vi "Overview Mouse Down.vi"(8 "error in":errorcluster, 10 "Coords":T1, 11 "XYGraphOverview in":refnum<class "XYGraphOverview.lvclass">) -> (0 "error out":errorcluster, 3 "XYGraphOverview out":refnum<class "XYGraphOverview.lvclass">)   [LabVIEW 2020, in "XYGraphOverview.lvlib" / "XYGraphOverview.lvclass"]
uses:
  XYGraphOverview.lvclass
  <vilib>/Utility/miscctls.llb/LVPoint32TypeDef.ctl
  XYGraphOverview.lvclass/XYGraphOverview.ctl
  Read Highlight Block Color.vi
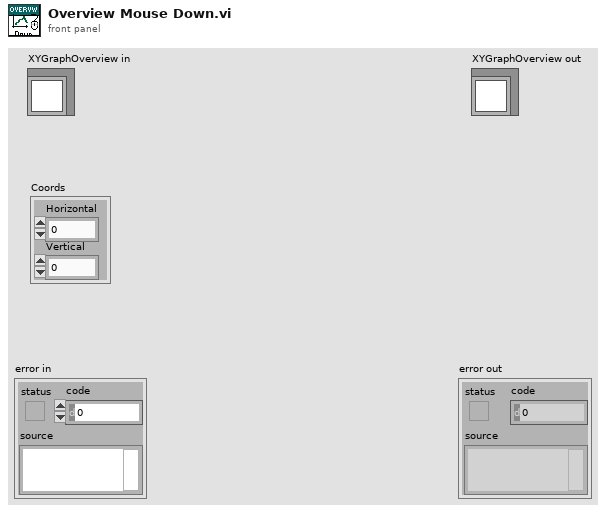
[diagram p1: front panel]
types:
  T1 = typedef "LVPoint32TypeDef.ctl" = cluster{"Horizontal":i32, "Vertical":i32}
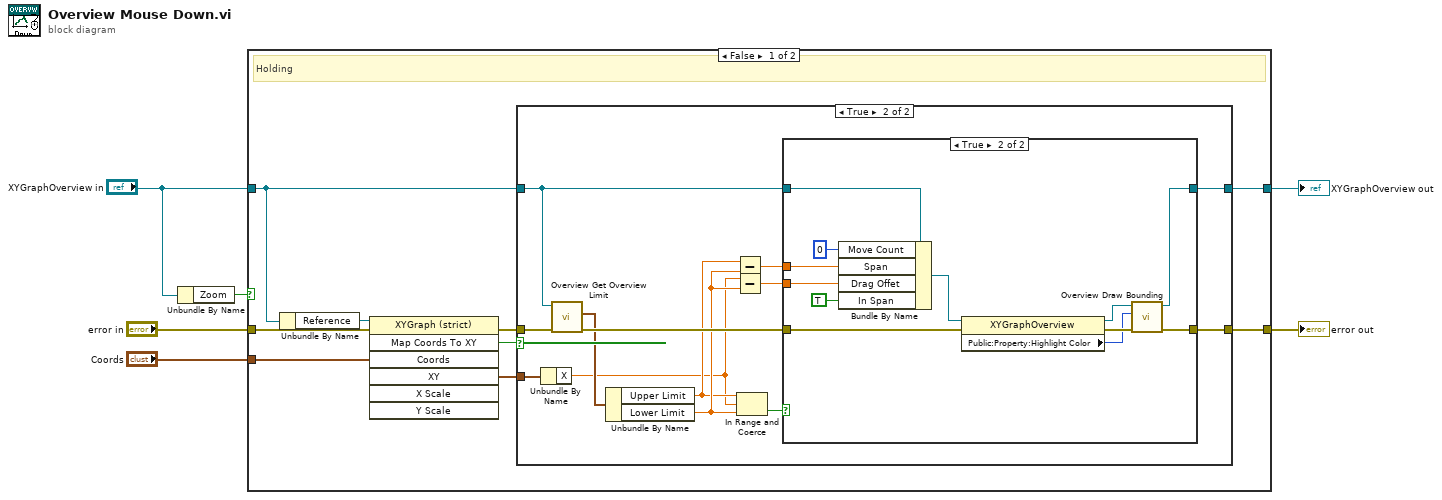
[diagram p0: block diagram]
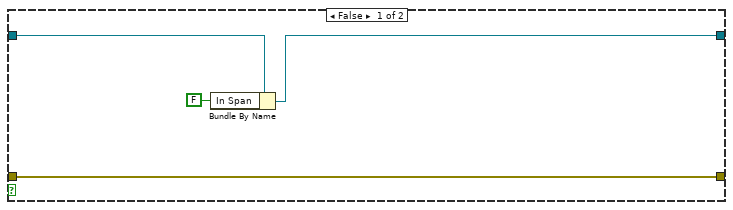
[diagram p2: hidden frame]
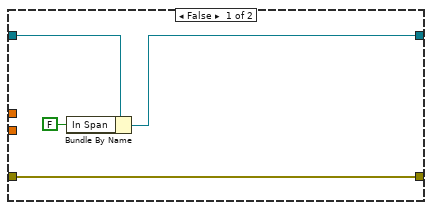
[diagram p3: hidden frame]
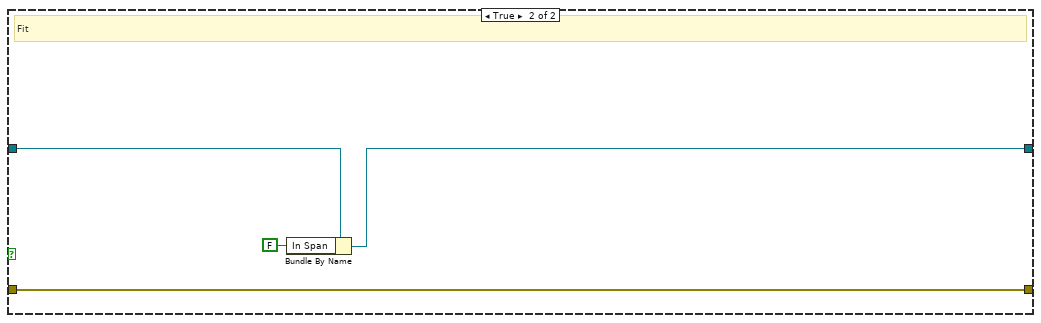
[diagram p4: hidden frame]
diagram:
  n1 = Unbundle By Name("XYGraphOverview in") -> ("Zoom"=w1:bool)
  n2 = case shown="False" w1 {
    tunnel: "Coords" -> [w15 _]
    tunnel: [w11 w52] -> w5
    tunnel: "error in" -> [w10 w52]
    tunnel: [w9 w49] -> w4
    tunnel: "XYGraphOverview in" -> [w8 w51]
    frame False {
      # "Holding"
      n3 = Unbundle By Name(w8) -> ("Reference"=w7:refnum<vi>)
      n4 = invoke on="Invoke Node" class="XYGraph (strict)" method="Map Coords To XY"(reference=w7, error in=w10, "Coords"=w15) -> (error out=w12:errorcluster, "Map Coords To XY"=w14:bool, "XY"=w13:cluster{"X":dbl, "Y":dbl})  [unwired: 4 in, 4 out]
      n5 = case shown="True" w14 {
        tunnel: w13 -> [_ w31]
        tunnel: w12 -> [w19 w28]
        tunnel: [w19 w32] -> w11
        tunnel: w8 -> [w18 w24]
        tunnel: [w16 w25] -> w9
        frame False {
          n6 = Bundle By Name(cluster=w18, "In Span"=FALSE) -> (w16:refnum<class "XYGraphOverview.lvclass">)
        }
        frame True {
          n7 = Unbundle By Name(w31) -> ("X"=w20:dbl)
          n8 = call "Overview Get Overview Limit.vi"("error in"=w28, "XYGraphOverview in"=w24) -> ("error out"=w27:errorcluster, "Limit"=w26:cluster{"Lower Limit":dbl, "Upper Limit":dbl})  [unwired: 7 in, 1 out]
          n9 = Unbundle By Name(w26) -> ("Upper Limit"=w21:dbl, "Lower Limit"=w23:dbl)
          n10 = Subtract(x=w21, y=w23) -> (x-y=w22:dbl)
          n11 = Subtract(x=w20, y=w23) -> (x-y=w29:dbl)
          n12 = In Range and Coerce(upper limit=w21, x=w20, lower limit=w23) -> (In Range?=w30:bool)  [unwired: 1 out]
          n13 = case shown="True" w30 {
            tunnel: w27 -> [w36 w40]
            tunnel: [w36 w38] -> w32
            tunnel: w29 -> [_ w47]
            tunnel: w24 -> [w35 w48]
            tunnel: [w33 w37] -> w25
            tunnel: w22 -> [_ w45]
            frame False {
              n14 = Bundle By Name(cluster=w35, "In Span"=FALSE) -> (w33:refnum<class "XYGraphOverview.lvclass">)
            }
            frame True {
              n15 = Bundle By Name(cluster=w48, "Move Count"=u32 0, "Span"=w45, "Drag Offet"=w47, "In Span"=TRUE) -> (w39:refnum<class "XYGraphOverview.lvclass">)
              n16 = property class="XYGraphOverview"(reference=w39, error in=w40) -> (reference out=w42:refnum<class "XYGraphOverview.lvclass">, error out=w43:errorcluster, "Public:Property:Highlight Color"=w41:u32)
              n17 = call "Overview Draw Bounding.vi"("error in (no error)"=w43, "Color"=w41, "XYGraphOverview in"=w42) -> ("error out"=w38:errorcluster, "XYGraphOverview out"=w37:refnum<class "XYGraphOverview.lvclass">)  [unwired: 7 in]
            }
          }
        }
      }
    }
    frame True {
      # "Fit"
      n18 = Bundle By Name(cluster=w51, "In Span"=FALSE) -> (w49:refnum<class "XYGraphOverview.lvclass">)
    }
  }
  "error out" <- w5
  "XYGraphOverview out" <- w4
